vi "Create File.vi"() -> ()   [LabVIEW 2017]
uses:
  Public/Controls/Version Info.ctl
  DSF Configuration API.lvlib
panel:
  out "names 2":string[](array[string])
  out "names":string[](array[string])
  out "version":T1
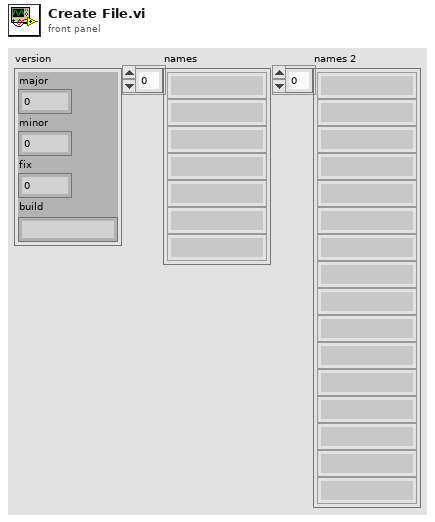
[diagram p1: front panel]
types:
  T1 = typedef "DSF Configuration API.lvlib/Version Info.ctl" = cluster{"major":u32, "minor":u32, "fix":u32, "build":string}
  T2 = typedef "DSF Configuration API.lvlib/DSF Config Data RefNum.ctl" = refnum<k1>
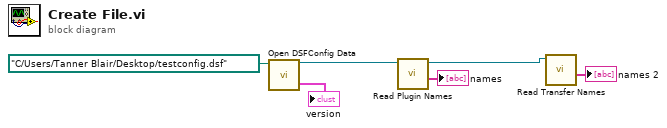
[diagram p0: block diagram]
diagram:
  n1 = call "Open DSFConfig Data.vi"("dsf configuration file path"=path "C:/Users/Tanner Blair/Desktop/testconfig.dsf") -> ("dsf refnum"=w4:T2, "version"=→"version":T1)  [unwired: 7 in, 2 out]
  n2 = call "Read Plugin Names.vi"("dsf refnum"=w4) -> ("names"=→"names":string[], "dsf refnum out"=w2:T2)  [unwired: 8 in, 1 out]
  n3 = call "Read Transfer Names.vi"("dsf refnum"=w2) -> ("names"=→"names 2":string[])  [unwired: 8 in, 2 out]
